vi "Channel Name.vi"(11 "Channel property":cluster{i32, "Channels":i32}[](array[cluster])) -> (3 "Channel Name":string[](array[string]))   [LabVIEW 2018]
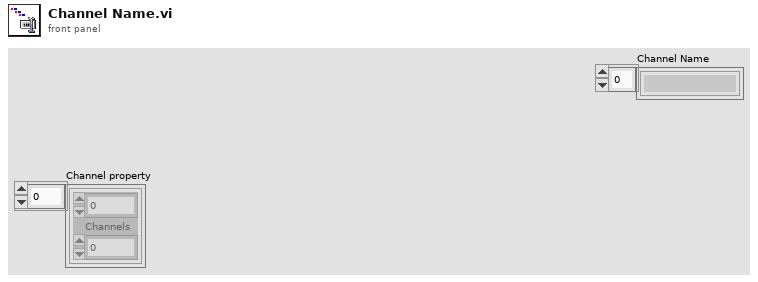
[diagram p1: front panel]
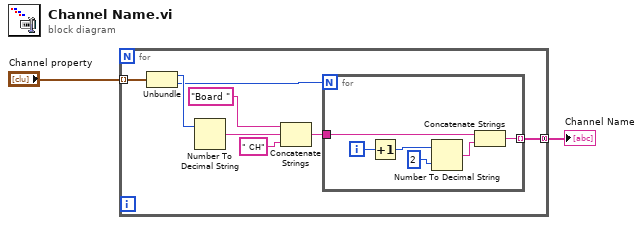
[diagram p0: block diagram]
diagram:
  n1 = for {
    tunnel: "Channel property" -> [w10] mode=indexing
    tunnel: [w3] -> w1 mode=concatenating
    n2 = Unbundle(w10) -> (w9:i32, "Channels"=w6:i32)
    n3 = Number To Decimal String(number=w9) -> (decimal integer string=w7:string)  [unwired: 1 in]
    n4 = Concatenate Strings("Board ", w7, " CH" ("string")) -> (w5:string)
    n5 = for {
      N: w6 -> [_]
      tunnel: w5 -> [w13]
      tunnel: [w11] -> w3 mode=indexing
      i -> [w16]
      n6 = Increment(x=w16) -> (x+1=w14:i32)
      n7 = Number To Decimal String(number=w14, width (-)=i16 2) -> (decimal integer string=w12:string)
      n8 = Concatenate Strings(w13, w12) -> (w11:string)
    }
  }
  "Channel Name" <- w1
